vi "StringConcatenate.vi"() -> ()   [LabVIEW 2019]
panel:
  in  "c":string="Pomogrenate"
  out "concatenated string":string
  in  "b":string="World"
  in  "a":string="Hello"
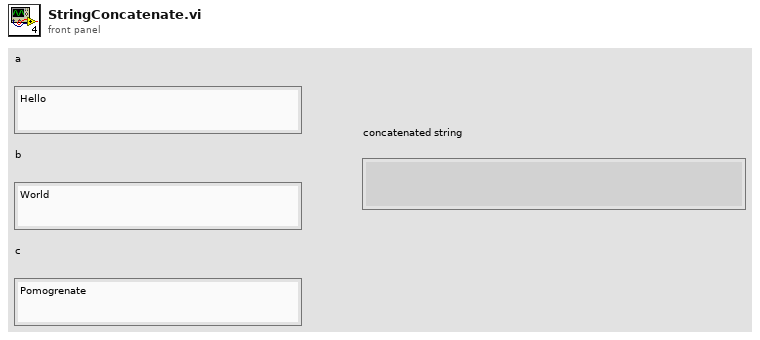
[diagram p1: front panel]
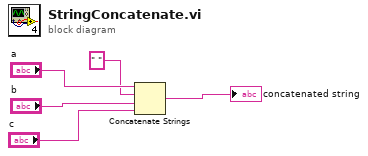
[diagram p0: block diagram]
diagram:
  n1 = Concatenate Strings("a", " " ("string"), "b", "c") -> (→"concatenated string":string)
